vi "Invert Direction.vi"(11 "Direction":T1) -> (3 "invert Direction":T1)   [LabVIEW 2019, in "Stand.lvclass"]
uses:
  Stand.lvclass
  TypeDef/Direction.ctl
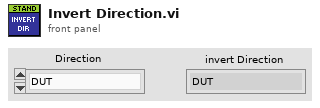
[diagram p1: front panel]
types:
  T1 = typedef "Direction.ctl" = enum8{"DUT", "Chamber"}
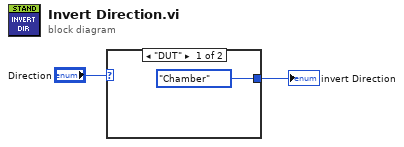
[diagram p0: block diagram]
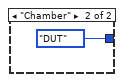
[diagram p2: hidden frame]
diagram:
  n1 = case shown="\"DUT\"" "Direction" {
    tunnel: [Direction."Chamber" ("Direction") Direction."DUT" ("Direction")] -> w2
    frame "DUT" {
    }
    frame "Chamber" {
    }
  }
  "invert Direction" <- w2
